vi "ReadGUID.vi"(0 "object in":refnum<class "Test2(ByValue).lvclass">, 5 "error in (no error)":errorcluster) -> (14 "object out":refnum<class "Test2(ByValue).lvclass">, 15 "GUID":string, 19 "error out":errorcluster)   [LabVIEW 2016, in "Test2(ByValue).lvclass"]
uses:
  Test2(ByValue).lvclass
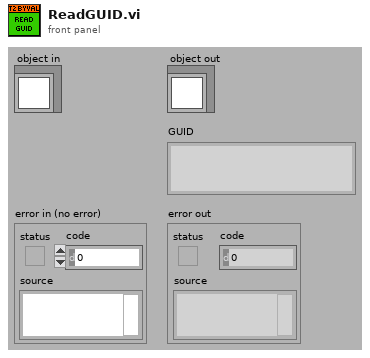
[diagram p1: front panel]
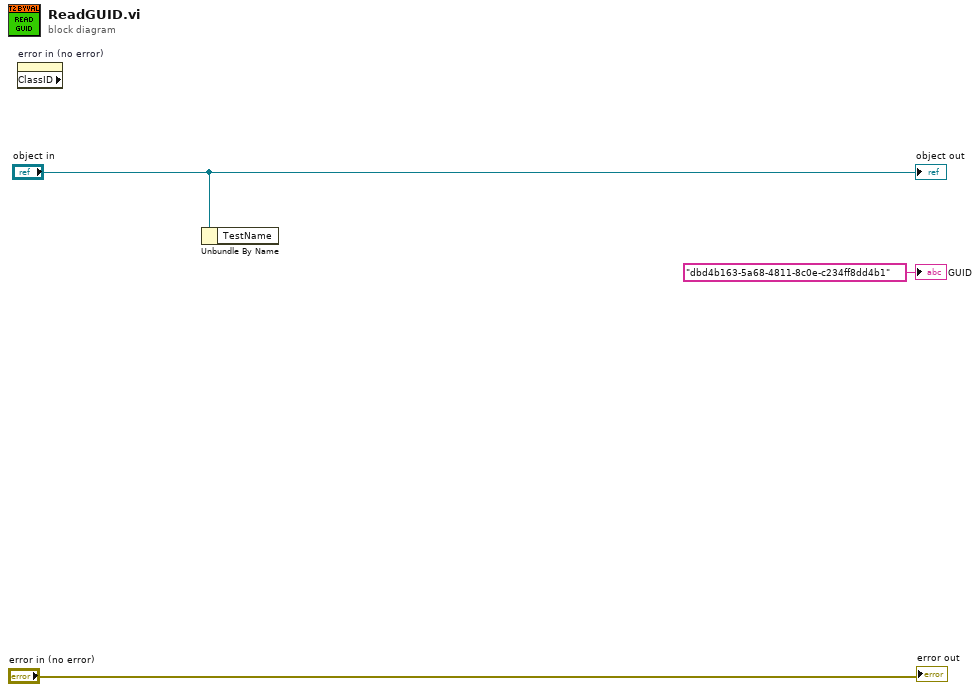
[diagram p0: block diagram]
diagram:
  n1 = property on="error in (no error)" class="Clust (strict)" props=["ClassID"]() -> ()  [unwired: 2 in, 3 out]
  n2 = Unbundle By Name("object in") -> ()  [unwired: 1 out]
  "error out" <- "error in (no error)"
  "object out" <- "object in"
  "GUID" <- "dbd4b163-5a68-4811-8c0e-c234ff8dd4b1" ("GUID")
